vi "Read Pigeon.vi"(11 "PigeonIMUDevRef":T1 {"Type" items=["CAN"=352321536, "TalonSRX"=33554432]}) -> (2 "Yaw":dbl)   [LabVIEW 2017]
uses:
  <vilib>/Rock Robotics/WPI/ThirdParty/Phoenix-LabVIEW/Pigeon IMU/CTRE_PigeonIMU_DeviceRef.ctl
  <vilib>/Rock Robotics/WPI/ThirdParty/Phoenix-LabVIEW/Pigeon IMU/CTRE_PigeonIMU_ConnectionType.ctl
  <vilib>/Rock Robotics/WPI/ThirdParty/Phoenix-LabVIEW/Pigeon IMU/CTRE_PigeonIMU_GetYPR.vi
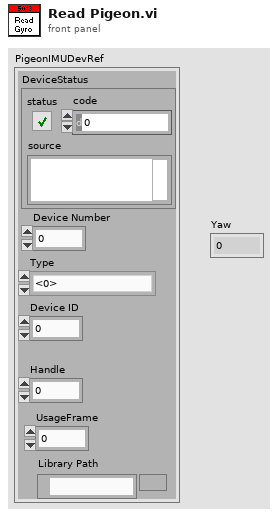
[diagram p1: front panel]
types:
  T1 = typedef "CTRE_PigeonIMU_DeviceRef.ctl" = cluster{"DeviceStatus":errorcluster, "Device Number":u8, "Type":T2, "Device ID":u32, "Handle":u64, "UsageFrame":u32, "Library Path":path}
  T2 = typedef "CTRE_PigeonIMU_ConnectionType.ctl" = u32
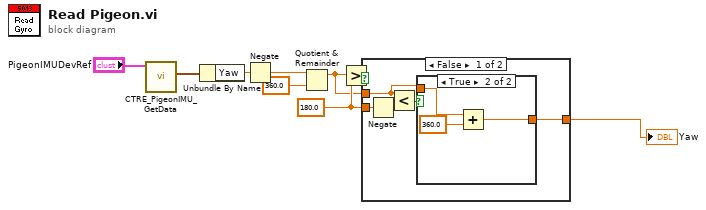
[diagram p0: block diagram]
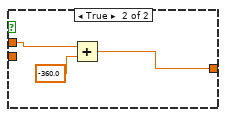
[diagram p3: hidden frame]
diagram:
  w9 = 180.0 ("y")
  n1 = call-poly <vilib>:"CTRE_PigeonIMU_GetData.vi"("PigeonIMUDevRef"="PigeonIMUDevRef") -> ("Yaw Pitch Roll"=w3:cluster{"Yaw":dbl, "Pitch":dbl, "Roll":dbl})  [unwired: 8 in, 2 out]
  n2 = Unbundle By Name(w3) -> ("Yaw"=w5:dbl)
  n3 = Negate(x=w5) -> (-x=w1:dbl)
  n4 = Quotient & Remainder(x=w1, y=360.0) -> (x-y*floor(x/y)=w8:dbl)  [unwired: 1 out]
  n5 = Greater?(x=w8, y=w9) -> (0:w7:bool)
  n6 = case shown="False" w7 {
    tunnel: w8 -> [w12 w20]
    tunnel: w9 -> [w11 _]
    tunnel: [w10 w19] -> w2
    frame False {
      n7 = Negate(x=w11) -> (-x=w13:dbl)
      n8 = Less?(x=w12, y=w13) -> (x < y?=w14:bool)
      n9 = case shown="True" w14 {
        tunnel: w12 -> [w15 w18]
        tunnel: [w15 w16] -> w10
        frame False {
        }
        frame True {
          n10 = Add(x=w18, y=360.0) -> (x+y=w16:dbl)
        }
      }
    }
    frame True {
      n11 = Add(x=w20, y=-360.0) -> (x+y=w19:dbl)
    }
  }
  "Yaw" <- w2
